vi "closestTack.vi"(8 "Irons Range":dbl=45.0, 9 "Absolute Wind Direction":dbl, 10 "Boat location":T1 {"North" format="%#_10f"; "East" format="%#_8f"}, 11 "PointA":T1 {"North" format="%#_10f"; "East" format="%#_8f"}) -> (3 "closest tack":dbl)   [LabVIEW 2013]
uses:
  Data/TypeDefs/UTM Location.ctl
panel:
  out "output  b":dbl format="%.2f"
  out "output a":dbl format="%.2f"
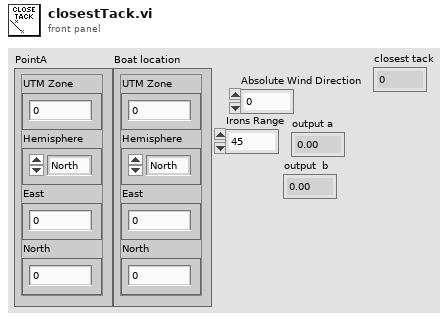
[diagram p1: front panel]
types:
  T1 = typedef "UTM Location.ctl" = cluster{"UTM Zone":dbl, "Hemisphere":enum16{"North", "South"}, "East":dbl, "North":dbl}
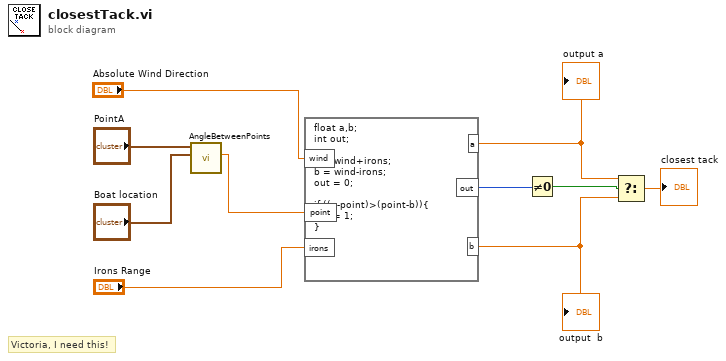
[diagram p0: block diagram]
diagram:
  # "Victoria, I need this!"
  n1 = call "AngleBetweenPoints.vi"("Point 2"="Boat location", "Point 1"="PointA") -> ("Angle"=w6:dbl)  [unwired: 9 in]
  n2 = formula code="float a,b;\nint out;\n\na = wind+irons;\nb = wind-irons;\nout = 0;\n\nif ((a-point)>(point-b)){\nout = 1;\n}"("wind"="Absolute Wind Direction", "irons"="Irons Range", "point"=w6) -> ("out"=w8:i32, "a"=w3:dbl, "b"=w2:dbl)
  "output a" <- w3
  "output  b" <- w2
  n3 = Not Equal To 0?(x=w8) -> (x != 0?=w4:bool)
  n4 = Select(t=w3, s=w4, f=w2) -> (s? t:f=→"closest tack":dbl)
